vi "SETPATHdll_Test.vi"(8 "error in (no error)":errorcluster) -> (0 "error out":errorcluster, 3 "Passed?":bool)   [LabVIEW 2021]
panel:
  out "hpath out":string
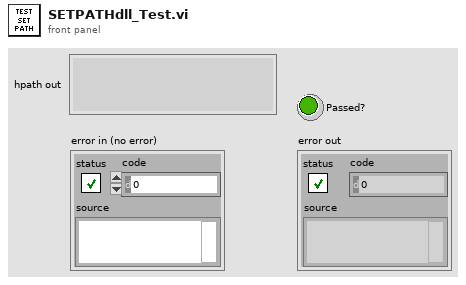
[diagram p1: front panel]
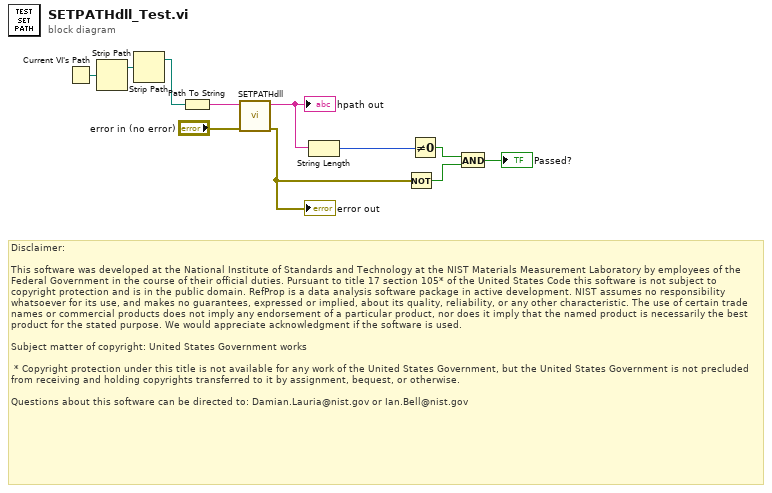
[diagram p0: block diagram]
diagram:
  # "Disclaimer:\n\nThis software was developed at the National Institute of Standards and Technology at the NIST Materials Measurement Laboratory by employees of the Federal Government in the course of their official duties. Pursuant to title 17 section 105* of the United States Code this software is not subject to copyright protection and is in the public domain. RefProp is a data analysis software package in active development. NIST assumes no responsibility whatsoever for its use, and makes no guarantees, expressed or implied, about its quality, reliability, or any other characteristic. The use of certain trade names or commercial products does not imply any endorsement of a particular product, nor does it imply that the named product is necessarily the best product for the stated purpose. We would appreciate acknowledgment if the software is used.\n \nSubject matter of copyright: United States Government works\n  \n * Copyright protection under this title is not available for any work of the United States Government, but the United States Government is not precluded from receiving and holding copyrights transferred to it by assignment, bequest, or otherwise.\n\nQuestions about this software can be directed to: Damian.Lauria@nist.gov or Ian.Bell@nist.gov"
  n1 = Current VI's Path() -> (path=w5:path)
  n2 = Strip Path(path=w5) -> (stripped path=w4:path)  [unwired: 1 out]
  n3 = Strip Path(path=w4) -> (stripped path=w3:path)  [unwired: 1 out]
  n4 = Path To String(path=w3) -> (string=w10:string)
  n5 = call "SETPATHdll.vi"("error in (no error)"="error in (no error)", "hpath"=w10) -> ("error out"=w9:errorcluster, "hpath out"=w2:string)  [unwired: 8 in]
  "error out" <- w9
  "hpath out" <- w2
  n6 = String Length(string=w2) -> (length=w1:i32)
  n7 = Not(x=w9) -> (.not. x?=w7:bool)
  n8 = Not Equal To 0?(x=w1) -> (x != 0?=w8:bool)
  n9 = And(x=w8, y=w7) -> (x .and. y?=→"Passed?":bool)
